vi "ConfigureMeasureRange.vi"(7 "SMU":T2, 8 "Error In":errorcluster, 9 "Range Function":T1, 10 "Measure Configuration":T3={"Enabled?"=FALSE, "Count"=1, "Interval (sec)"=0.025, "Voltage Auto Range Enabled?"=TRUE, "Voltage High Limit (V or A)"=0.0, "Voltage Low Limit (V or A)"=0.0, "Current Auto Range Enabled?"=TRUE, "Current High Limit (V or A)"=0.0, "Current Low Limit (V or A)"=0.0} {"Count" min=1 step=1}, 11 "Keithley 2602 In":refnum<visa-resource-name>) -> (0 "Error Out":errorcluster, 3 "Keithley 2602 Out":refnum<visa-resource-name>)   [LabVIEW 2012]
uses:
  MeasureConfiguration.ctl
  driver/Public/Controls/SMU.ctl
  driver/Public/Controls/RangeFunction.ctl
  driver/Keithley-2602.lvlib
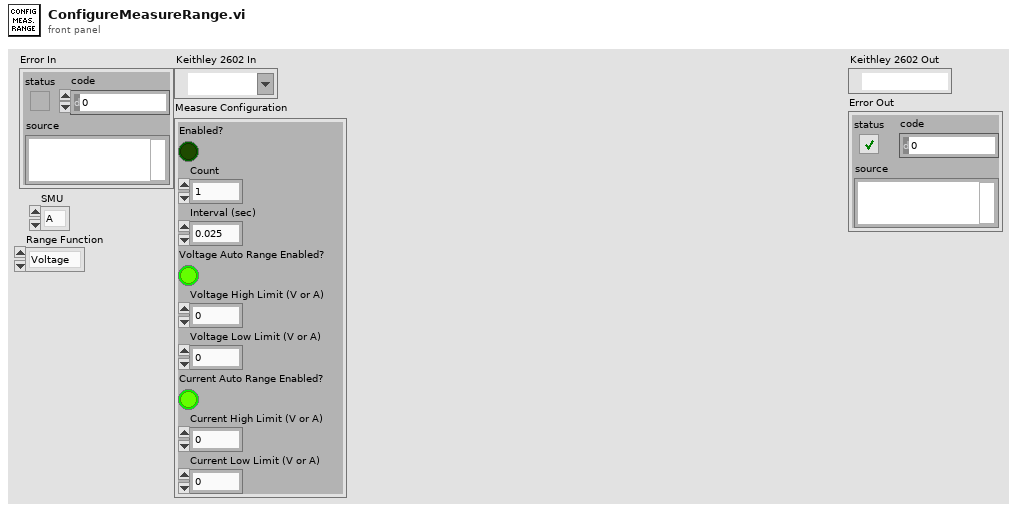
[diagram p1: front panel]
types:
  T1 = typedef "Keithley-2602.lvlib/RangeFunction.ctl" = enum16{"Voltage", "Current"}
  T2 = typedef "Keithley-2602.lvlib/SMU.ctl" = enum16{"A", "B"}
  T3 = typedef "MeasureConfiguration.ctl" = cluster{"Enabled?":bool, "Count":u8, "Interval (sec)":dbl, "Voltage Auto Range Enabled?":bool, "Voltage High Limit (V or A)":dbl, "Voltage Low Limit (V or A)":dbl, "Current Auto Range Enabled?":bool, "Current High Limit (V or A)":dbl, "Current Low Limit (V or A)":dbl}
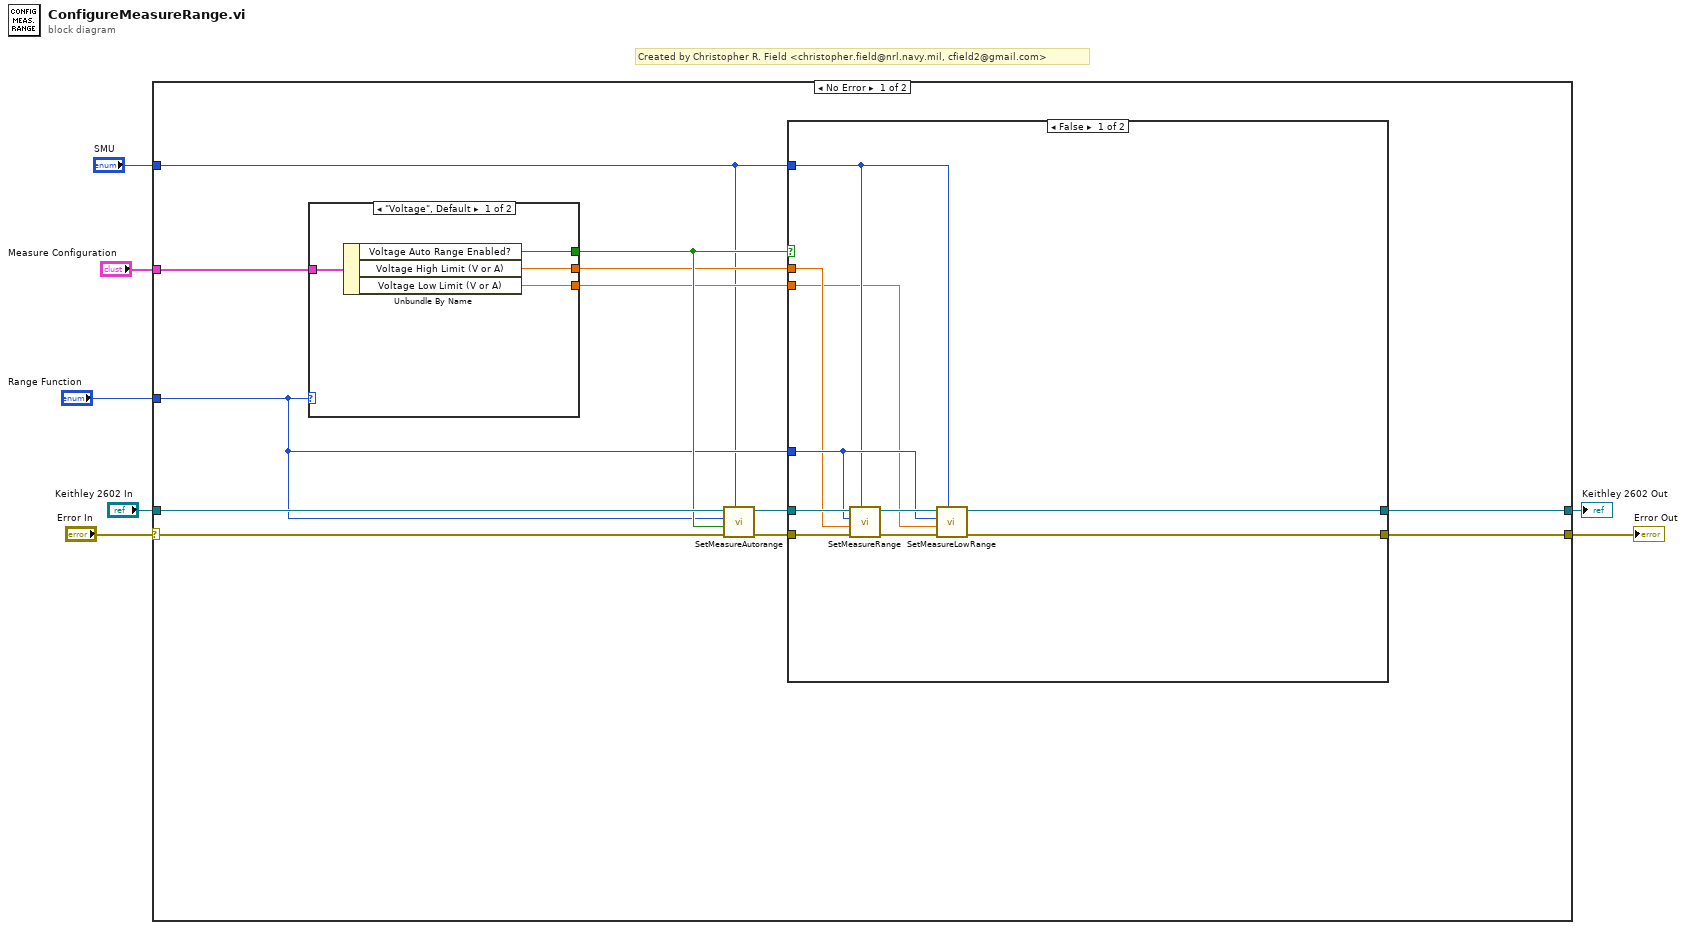
[diagram p0: block diagram]
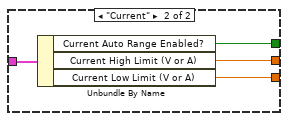
[diagram p2: hidden frame]
diagram:
  # "Created by Christopher R. Field <christopher.field@nrl.navy.mil, cfield2@gmail.com>"
  n1 = case shown="No Error" "Error In" {
    selector: "Error In" -> [w17 w40]
    tunnel: "Keithley 2602 In" -> [w16 w41]
    tunnel: "Measure Configuration" -> [w15 _]
    tunnel: "SMU" -> [w10 _]
    tunnel: "Range Function" -> [w11 _]
    tunnel: [w9 w41] -> w2
    tunnel: [w8 w40] -> w1
    frame No Error {
      n2 = case shown="\"Voltage\", Default" w11 {
        tunnel: w15 -> [w23 w27]
        tunnel: [w22 w26] -> w14
        tunnel: [w21 w25] -> w13
        tunnel: [w20 w24] -> w12
        frame "Voltage", Default {
          n3 = Unbundle By Name(w23) -> ("Voltage Auto Range Enabled?"=w22:bool, "Voltage High Limit (V or A)"=w21:dbl, "Voltage Low Limit (V or A)"=w20:dbl)
        }
        frame "Current" {
          n4 = Unbundle By Name(w27) -> ("Current Auto Range Enabled?"=w26:bool, "Current High Limit (V or A)"=w25:dbl, "Current Low Limit (V or A)"=w24:dbl)
        }
      }
      n5 = call "SetMeasureAutorange.vi"("SMU"=w10, "Error In"=w17, "Enable?"=w14, "Range Function"=w11, "Keithley 2602 In"=w16) -> ("Error Out"=w18:errorcluster, "Keithley 2602 Out"=w19:refnum<visa-resource-name>)  [unwired: 5 in]
      n6 = case shown="False" w14 {
        tunnel: w19 -> [w37 w39]
        tunnel: w18 -> [w36 w38]
        tunnel: [w33 w39] -> w9
        tunnel: [w32 w38] -> w8
        tunnel: w13 -> [w29 _]
        tunnel: w12 -> [w28 _]
        tunnel: w11 -> [w31 _]
        tunnel: w10 -> [w30 _]
        frame False {
          n7 = call "SetMeasureRange.vi"("SMU"=w30, "Error In"=w36, "Range (V or A)"=w29, "Range Function"=w31, "Keithley 2602 In"=w37) -> ("Error Out"=w34:errorcluster, "Keithley 2602 Out"=w35:refnum<visa-resource-name>)  [unwired: 5 in]
          n8 = call "SetMeasureLowRange.vi"("SMU"=w30, "Error In"=w34, "Range (V or A)"=w28, "Range Function"=w31, "Keithley 2602 In"=w35) -> ("Error Out"=w32:errorcluster, "Keithley 2602 Out"=w33:refnum<visa-resource-name>)  [unwired: 5 in]
        }
        frame True {
        }
      }
    }
    frame Error {
    }
  }
  "Keithley 2602 Out" <- w2
  "Error Out" <- w1
